vi "Host - Get Local and ECAT Masters.vi"(8 "error in (no error)":errorcluster, 11 "Refnum in":refnum<k21>) -> (0 "error out":errorcluster, 1 "Local UDV Container":refnum<k21>[](array[refnum]), 2 "All Local Mods":refnum<k21>[](array[refnum]), 3 "All ECAT Masters":refnum<k21>[](array[refnum]))   [LabVIEW 2019, in "Scan Engine Custom Device.lvlib"]
uses:
  Scan Engine Custom Device.lvlib
  <resource>/objmgr/ni.var.rc
panel:
  out "XMLPfad":path
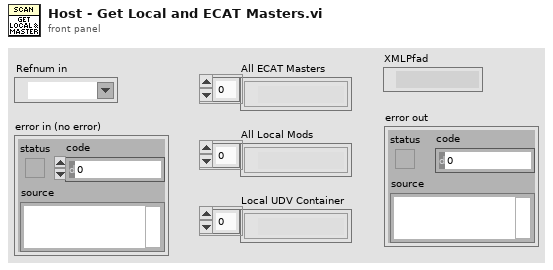
[diagram p1: front panel]
types:
  T1 = enum16{"open", "replace", "create", "open or create", "replace or create", "replace or create with confirmation"}
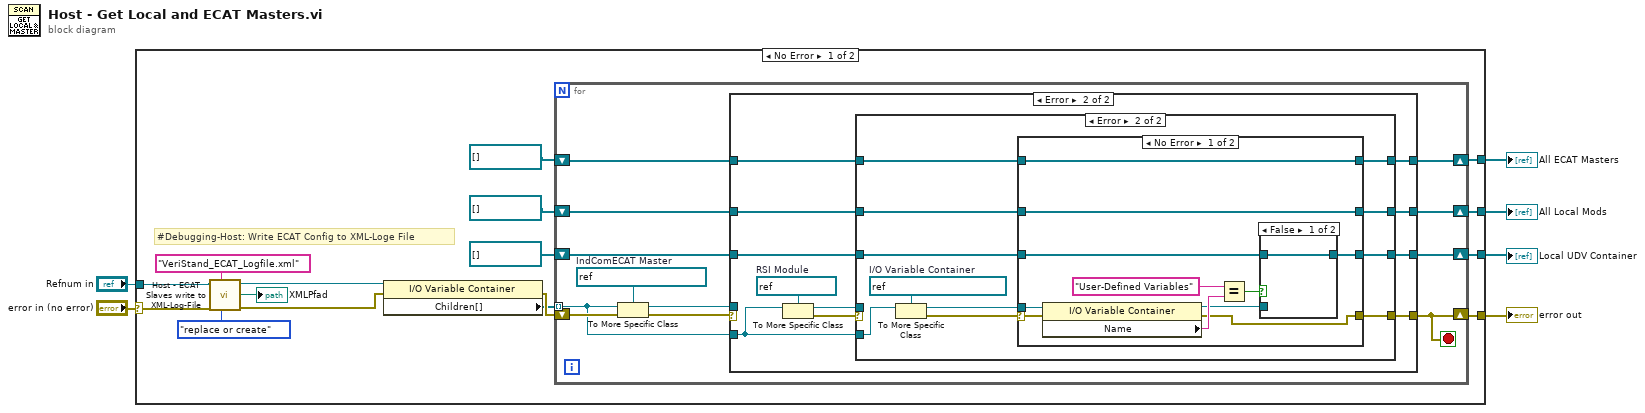
[diagram p0: block diagram]
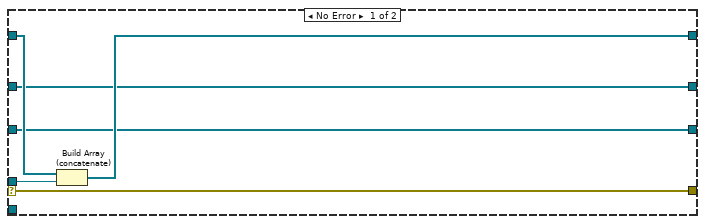
[diagram p2: hidden frame]
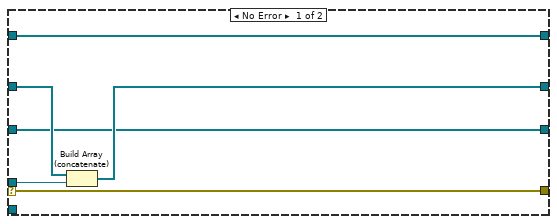
[diagram p3: hidden frame]
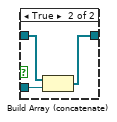
[diagram p4: hidden frame]
diagram:
  n1 = case shown="No Error" "error in (no error)" {
    selector: "error in (no error)" -> [w12 w88]
    tunnel: "Refnum in" -> [w13 _]
    tunnel: [w22 _] -> w5
    tunnel: [w21 _] -> w4
    tunnel: [w20 _] -> w3
    tunnel: [w14 w88] -> w2
    frame No Error {
      # "#Debugging-Host: Write ECAT Config to XML-Loge File"
      n2 = call "Host - ECAT Slaves write to XML-Log-File.vi"("Operation (0:Öffnen)"=T1."replace or create", "XML Log File name"="VeriStand_ECAT_Logfile.xml" ("name or relative path"), "Fehler (Eingang, kein Fehler)"=w12, "Referenz (Eingang)"=w13) -> ("Fehler (Ausgang)"=w10:errorcluster, "Pfad"=→"XMLPfad":path, "Referenz (Ausgang)"=w11:refnum<k21>)  [unwired: 5 in]
      n3 = property class="I/O Variable Container"(reference=w11, error in=w10) -> (error out=w19:errorcluster, "Children[]"=w18:refnum<k21>[])  [unwired: 1 out]
      n4 = for {
        tunnel: w18 -> [w28] mode=indexing
        shift-right: [w30] -> w22
        shift-left: refnum<k21>[] [] -> [w29]
        shift-right: [w26] -> w20
        shift-left: refnum<k21>[] [] -> [w27]
        shift-right: [w24] -> w21
        shift-left: refnum<k21>[] [] -> [w25]
        shift-right: [w23] -> w14
        shift-left: w19 -> [w34]
        stop <- w23 stop-if-true
        w33 = refnum<k21> refnum  # IndComECAT Master
        n5 = To More Specific Class(target class=w33, reference=w28, error in=w34) -> (specific class reference=w31:refnum<k21>, error out=w32:errorcluster)
        n6 = case shown="Error" w32 {
          selector: w32 -> [w38 _]
          tunnel: w31 -> [w35 _]
          tunnel: [w40 w45] -> w30
          tunnel: w29 -> [w39 w46]
          tunnel: [w38 w44] -> w23
          tunnel: w28 -> [_ w43]
          tunnel: w27 -> [w37 w48]
          tunnel: [w37 w47] -> w26
          tunnel: w25 -> [w36 w42]
          tunnel: [w36 w41] -> w24
          frame No Error {
            n7 = Build Array (concatenate)(w39, w35) -> (w40:refnum<k21>[])
          }
          frame Error {
            w51 = refnum<k21> refnum  # RSI Module
            n8 = To More Specific Class(target class=w51, reference=w43) -> (specific class reference=w49:refnum<k21>, error out=w50:errorcluster)  [unwired: 1 in]
            n9 = case shown="Error" w50 {
              tunnel: w49 -> [w53 _]
              selector: w50 -> [w52 _]
              tunnel: w48 -> [w57 w64]
              tunnel: [w56 w61] -> w47
              tunnel: w46 -> [w55 w63]
              tunnel: [w55 w62] -> w45
              tunnel: [w52 w58] -> w44
              tunnel: w43 -> [_ w67]
              tunnel: w42 -> [w54 w65]
              tunnel: [w54 w60] -> w41
              frame No Error {
                n10 = Build Array (concatenate)(w57, w53) -> (w56:refnum<k21>[])
              }
              frame Error {
                w68 = refnum<k21> refnum  # I/O Variable Container
                n11 = To More Specific Class(target class=w68, reference=w67) -> (specific class reference=w59:refnum<k21>, error out=w66:errorcluster)  [unwired: 1 in]
                n12 = case shown="No Error" w66 {
                  selector: w66 -> [w77 w84]
                  tunnel: w65 -> [w71 w87]
                  tunnel: w64 -> [w78 w86]
                  tunnel: w63 -> [w79 w85]
                  tunnel: [w79 w85] -> w62
                  tunnel: [w78 w86] -> w61
                  tunnel: [w70 w87] -> w60
                  tunnel: w59 -> [w76 _]
                  tunnel: [w69 w84] -> w58
                  frame No Error {
                    n13 = property class="I/O Variable Container"(reference=w76, error in=w77) -> (reference out=w72:refnum<k21>, error out=w69:errorcluster, "Name"=w75:string)
                    n14 = Equal?(x="User-Defined Variables", y=w75) -> (x = y?=w73:bool)
                    n15 = case shown="False" w73 {
                      tunnel: w72 -> [_ w82]
                      tunnel: w71 -> [w80 w83]
                      tunnel: [w80 w81] -> w70
                      frame False {
                      }
                      frame True {
                        n16 = Build Array (concatenate)(w83, w82) -> (w81:refnum<k21>[])
                      }
                    }
                  }
                  frame Error {
                  }
                }
              }
            }
          }
        }
      }
    }
    frame Error {
    }
  }
  "All ECAT Masters" <- w5
  "Local UDV Container" <- w4
  "All Local Mods" <- w3
  "error out" <- w2
